vi "S&E Debug string.vi"(2 "Elevated priority":bool, 5 "Type":variant, 7 "Content":variant, 9 "error in":errorcluster) -> (8 "Note":string, 10 "error out":errorcluster)   [LabVIEW 2011]
uses:
  emi Lib/System 01/0 - General/S&E reporting/Private/_emi_ S&E Message note.ctl
  <vilib>/Utility/VariantDataType/GetNumericInfo.vi
  <vilib>/Utility/VariantDataType/VariantType.lvlib
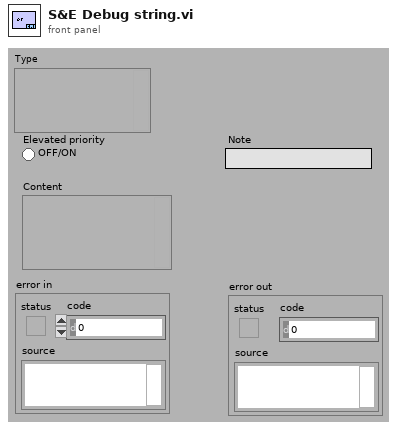
[diagram p1: front panel]
types:
  T1 = typedef "_emi_ S&E Message note.ctl" = cluster{"Note ID":i16, "Note":string}
  T2 = typedef "VariantType.lvlib/Type.ctl" = enum8{"Invalid Type", "Void", "I8", "I16", "I32", "I64", "U8", "U16", "U32", "U64", "Single Float", "Double Float", "Extended Float", "Single Complex", "Double Complex", "Extended Complex", "Enum U8", "Enum U16", "Enum U32", "Enum U64", "Single Float With Unit", "Double Float With Unit", "Extended Float With Unit", "Single Complex with Unit", "Double Complex with Unit", "Extended Complex with Unit", "Boolean", "String", "Path", "Picture", "Tag", "Array", "Cluster", "Variant", "LV Variant", "Waveform", "Timestamp", "Digital Waveform", "Digital Data", "ExpressData", "Refnum", "External Data", "VI", "Poly VI", "LabVIEW Class Instance", "Fixed Point"}
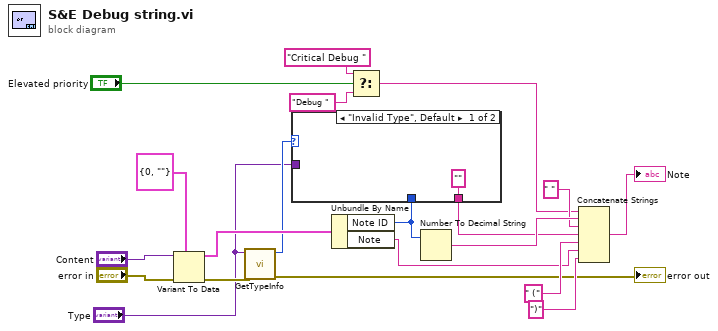
[diagram p0: block diagram]
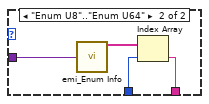
[diagram p2: hidden frame]
diagram:
  n1 = Variant To Data(error in="error in", type=T1 {"Note ID"=0, "Note"=""} ("E&S Note"), Variant="Content") -> (data=w7:T1, error out=w4:errorcluster)
  n2 = call <vilib>:"GetTypeInfo.vi"("error in (no error)"=w4, "Variant"="Type") -> ("error out"=→"error out":errorcluster, "Type Enum"=w2:T2)  [unwired: 5 in, 3 out]
  n3 = Unbundle By Name(w7) -> ("Note ID"=w14:i16, "Note"=w8:string)
  n4 = case shown="\"Invalid Type\", Default" w2 {
    tunnel: w14 -> [_ w24]
    tunnel: ["" ("String") w23] -> w11
    tunnel: "Type" -> [_ w22]
    frame "Invalid Type", Default {
    }
    frame "Enum U8".."Enum U64" {
      n5 = call "emi_Enum Info.vi"("Enum"=w22) -> ("Text Elements"=w25:string[])  [unwired: 11 in, 3 out]
      n6 = Index Array(array=w25, index=w24) -> (element=w23:string)
    }
  }
  n7 = Select(t="Critical Debug ", s="Elevated priority", f="Debug " ("format string")) -> (s? t:f=w5:string)
  n8 = Number To Decimal String(number=w14) -> (decimal integer string=w13:string)  [unwired: 1 in]
  n9 = Concatenate Strings(w5, w13, " " ("string"), w11, " (" ("string"), w8, ")" ("string")) -> (→"Note":string)
